vi "GetQ_single string.vi"(8 "error in (no error)":errorcluster, 10 "QName":string) -> (0 "error out":errorcluster, 1 "found":bool, 2 "Queue":refnum<queue>)   [LabVIEW 2020, in "QDict.lvlib"]
doc: "Developed by Kevin Thompson\nkevin@thompsonengineering.net\n\nCopyright 2021\nThompson Engineering, LLC"
uses:
  QDict.lvlib
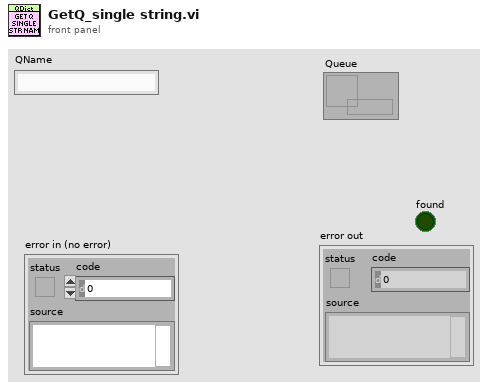
[diagram p1: front panel]
types:
  T1 = typedef "TD Dynamic CVT DVR--ref.ctl" = refnum<data-value>
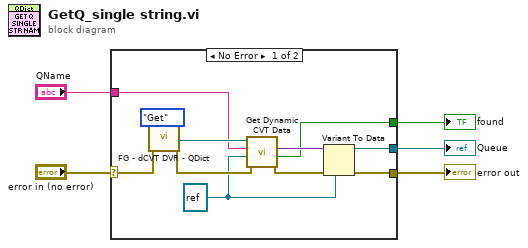
[diagram p0: block diagram]
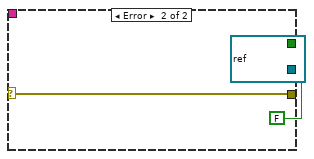
[diagram p2: hidden frame]
diagram:
  n1 = case shown="No Error" "error in (no error)" {
    selector: "error in (no error)" -> [w15 w19]
    tunnel: [w8 w19] -> w5
    tunnel: "QName" -> [w10 _]
    tunnel: [w9 refnum<queue> refnum ("queue out")] -> w2
    tunnel: [w7 FALSE ("found")] -> w1
    frame No Error {
      w6 = refnum<queue> refnum ("queue out")
      n2 = call "FG - dCVT DVR - QDict.vi"("error in (no error)"=w15, "Action (Get)"=enum16{"Init", "Get", "Set"}."Get") -> ("dCVT QMH out"=w14:T1, "error out"=w13:errorcluster)  [unwired: 7 in]
      n3 = call <vilib>:"Get Dynamic CVT Data.vi"("error in (no error)"=w13, "default value (empty variant)"=w6, "DataName"=w10, "dCVT DVR"=w14) -> ("error out"=w12:errorcluster, "found"=w7:bool, "value"=w11:variant)  [unwired: 4 in, 1 out]
      n4 = Variant To Data(error in=w12, type=w6, Variant=w11) -> (data=w9:refnum<queue>, error out=w8:errorcluster)
    }
    frame Error {
    }
  }
  "error out" <- w5
  "Queue" <- w2
  "found" <- w1
